vi "Shooter Controller.vi"(8 "error in":errorcluster) -> ()   [LabVIEW 2019]
doc: "This VI executes continuously carrying out the current operation and responding to updates or new operations. It will often contain the timing or control code that is difficult to place directly in TeleOp. This VI generally opens all sensors and motors and isolates the rest of the robot code from knowing how the operations are carried out."
uses:
  <vilib>/Rock Robotics/WPI/Framework/Completion Status.ctl
  Shooter Setpoints.ctl
  Shooter Operations.ctl
  <vilib>/Rock Robotics/WPI/ThirdParty/REV Robotics/SPARK MAX/Typedef/Spark MAX Idle Mode.ctl
  <vilib>/Rock Robotics/WPI/ThirdParty/REV Robotics/SPARK MAX/Typedef/Spark MAX Control Type.ctl
  <vilib>/Rock Robotics/Network Tables/NT Write Boolean.vi
panel:
  in  "Interactive Values":T1
  out "Current\nCmd":string
  in  "Buttons":cluster{"Execute Cmd":bool, "Abort Cmd":bool}
  out "Command Timing":cluster{"Start Time (ms)":u32, "Iterations":i32}
  out "Status":T3
  # "Tip: It may be helpful to observe inputs and sensor values.\nYou may also want to display tuning or debugging controls."
  # "Interactive Command: You may fill in the settings for a command\nand schedule it with the Execute button. You can observe and abort\nany command while fine tuning the code for the controller."
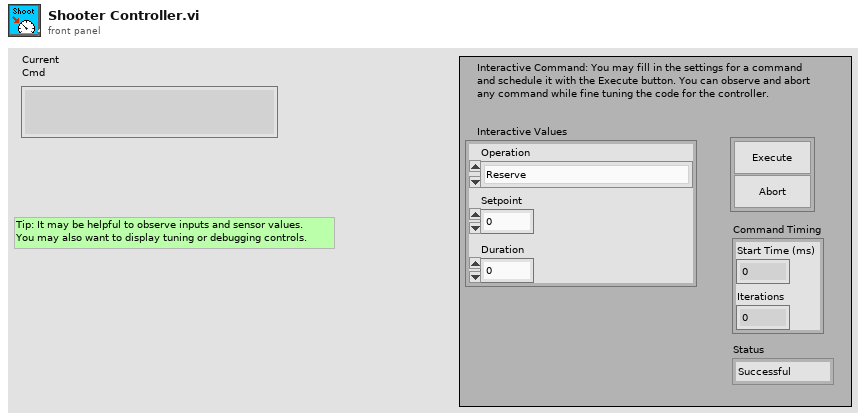
[diagram p1: front panel]
types:
  T1 = typedef "Shooter Setpoints.ctl" = cluster{"Operation":T2, "Setpoint":dbl, "Duration":dbl}
  T2 = typedef "Shooter Operations.ctl" = enum16{"Reserve", "Read Current", "Immediate", "Shoot for Time"}
  T3 = typedef "Completion Status.ctl" = enum16{"Successful", "Aborted", "Incomplete"}
  T4 = typedef "Spark MAX Idle Mode.ctl" = enum16{"Coast", "Brake"}
  T5 = typedef "WPI_MotorControlDeviceRef.ctl" = cluster{"DeviceStatus":errorcluster, "Type":T6, "PWM":cluster{"PWM Channel":T7, "DeadBand":T8}, "CAN":cluster{"Device Number":u8, "SetOutput VI Ref":variant, "GetOutput VI Ref":variant, "Enable VI Ref":variant, "Disable VI Ref":variant, "Data":variant}, "Invert":bool, "DIO PWM":cluster{"PWM \"Enable\" Channel":T7, "DIOChannel":T9, "PWM Rate":dbl}}
  T6 = typedef "WPI_MotorControlType.ctl" = enum16{"PWM", "CAN", "DIO PWM"}
  T7 = typedef "FPGA_DIOPWMChannel.ctl" = enum8{"PWM 0", "PWM 1", "PWM 2", "PWM 3", "PWM 4", "PWM 5", "PWM 6", "PWM 7", "PWM 8", "PWM 9", "PWM MXP 0", "PWM MXP 1", "PWM MXP 2", "PWM MXP 3", "PWM MXP 4", "PWM MXP 5", "PWM MXP 6", "PWM MXP 7", "PWM MXP 8", "PWM MXP 9", "Invalid"}
  T8 = typedef "WPI_PWMDeadband.ctl" = cluster{"Name":string, "maxPositivePwm":i32, "minPositivePwm":i32, "centerPwm":i32, "maxNegativePwm":i32, "minNegativePwm":i32, "angularRange":u16}
  T9 = typedef "FPGA_DIOChannel.ctl" = enum8{"DIO 0", "DIO 1", "DIO 2", "DIO 3", "DIO 4", "DIO 5", "DIO 6", "DIO 7", "DIO 8", "DIO 9", "DIO MXP 0", "DIO MXP 1", "DIO MXP 2", "DIO MXP 3", "DIO MXP 4", "DIO MXP 5", "DIO MXP 6", "DIO MXP 7", "DIO MXP 8", "DIO MXP 9", "DIO MXP 10", "DIO MXP 11", "DIO MXP 12", "DIO MXP 13", "DIO MXP 14", "DIO MXP 15", "SPI Port CS1", "SPI Port CS2", "SPI Port CS3", "SPI Port MISO", "SPI Port MOSI", "Invalid"}
  T10 = typedef "Command Status Info.ctl" = cluster{"Name":string, "Status":T3, "notifier out":T11}
  T11 = typedef "Completion Notifier.ctl" = refnum<notifier>
  T12 = cluster{"Current Command":T1, "Command Timing":cluster{"Start Time (ms)":u32, "Iterations":i32}, "Command Arguments":cluster{"Command Info":T10, "Description":string, "Default Command":T1, "queue out":refnum<queue>, "Subsystem Name":string}}
  T13 = typedef "Spark MAX Control Type.ctl" = enum16{"Percent VBus", "Voltage", "Velocity", "Position", "Smart Motion", "Current", "Smart Velocity"}
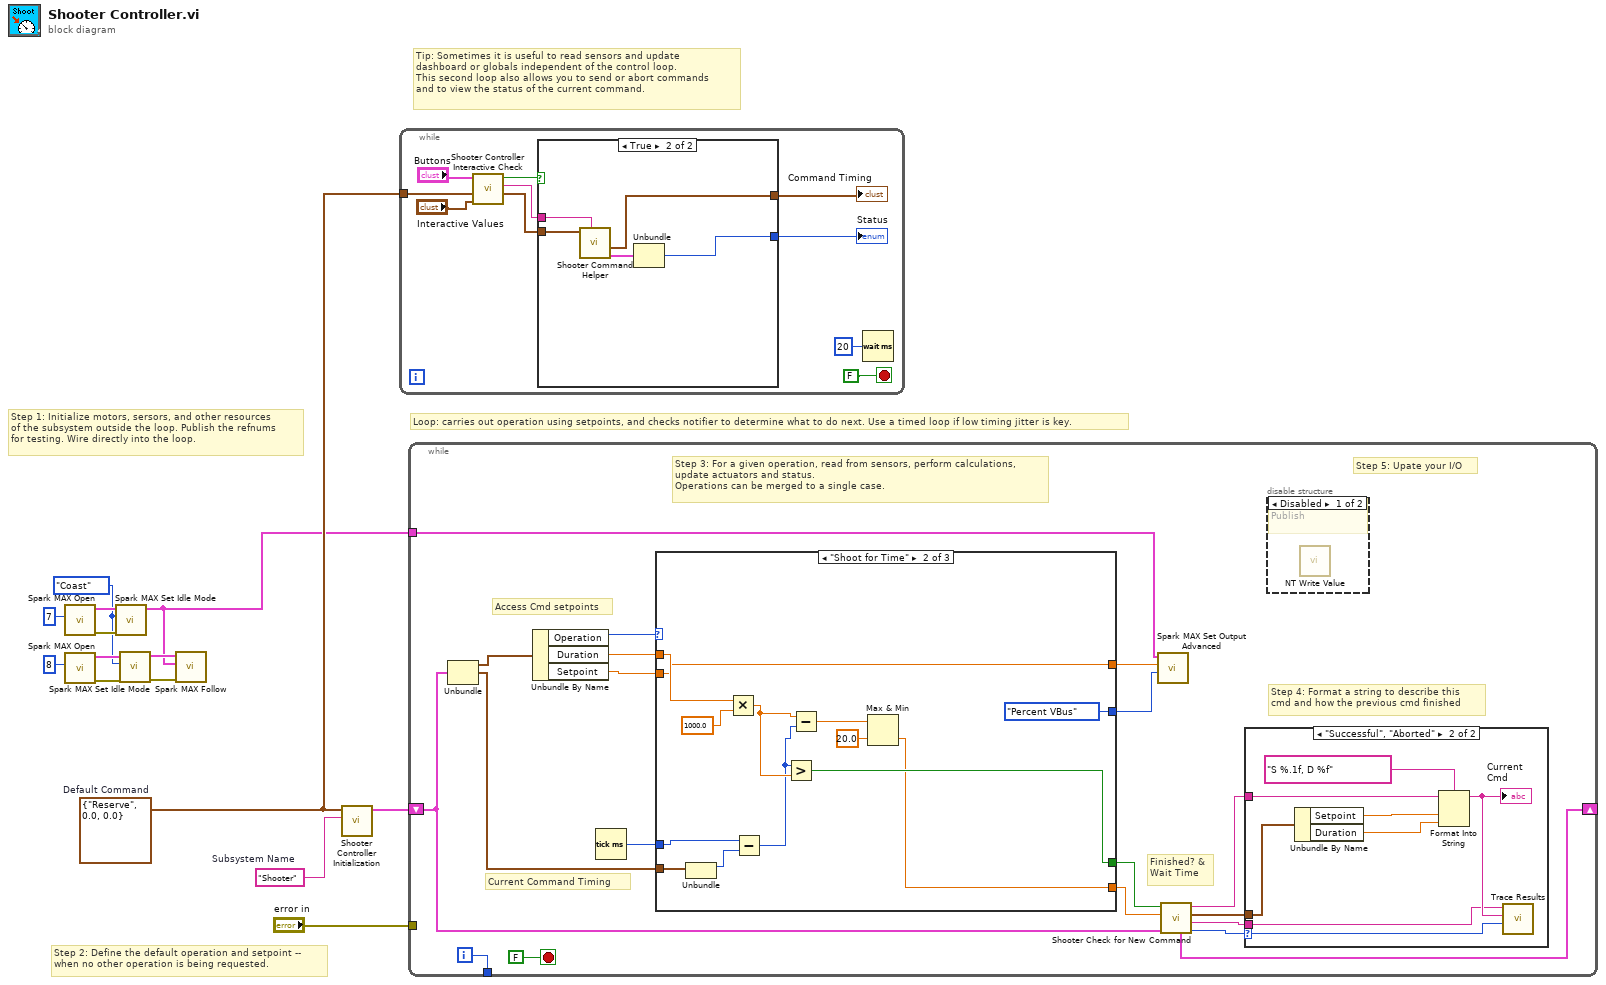
[diagram p0: block diagram]
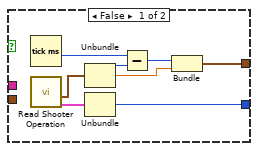
[diagram p2: hidden frame]
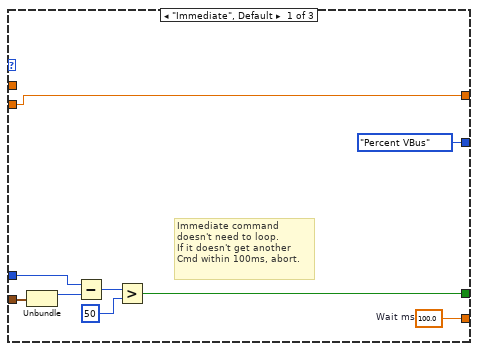
[diagram p5: hidden frame]
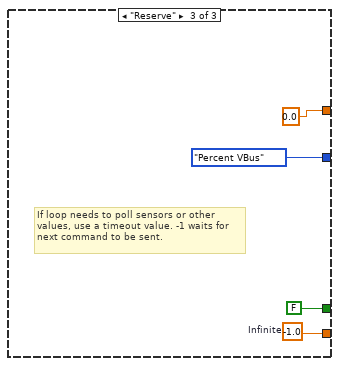
[diagram p6: hidden frame]
diagram:
  w6 = Spark_MAX_Idle_Mode."Coast" ("Idle Mode")
  w11 = T1 {"Operation"=enum."Reserve", "Setpoint"=0.0, "Duration"=0.0}  # Default Command
  w12 = "Shooter"  # Subsystem Name
  # "Tip: Sometimes it is useful to read sensors and update\ndashboard or globals independent of the control loop.\nThis second loop also allows you to send or abort commands\nand to view the status of the current command."
  # "Step 2: Define the default operation and setpoint --\nwhen no other operation is being requested."
  # "Step 1: Initialize motors, sersors, and other resources\nof the subsystem outside the loop. Publish the refnums\nfor testing. Wire directly into the loop."
  # "Loop: carries out operation using setpoints, and checks notifier to determine what to do next. Use a timed loop if low timing jitter is key."
  n1 = call <vilib>:"Spark MAX Open.vi"("Device Number"=u8 7) -> ("error out"=w10:errorcluster, "MotorControlDeviceRef"=w9:T5)  [unwired: 9 in]
  n2 = call <vilib>:"Spark MAX Open.vi"("Device Number"=u8 8) -> ("error out"=w7:errorcluster, "MotorControlDeviceRef"=w8:T5)  [unwired: 9 in]
  n3 = call <vilib>:"Spark MAX Set Idle Mode.vi"("error in (no error)"=w10, "Idle Mode"=w6, "MotorControlDeviceRef in"=w9) -> ("MotorControlDeviceRef out"=w1:T5)  [unwired: 7 in, 1 out]
  n4 = call <vilib>:"Spark MAX Set Idle Mode.vi"("error in (no error)"=w7, "Idle Mode"=w6, "MotorControlDeviceRef in"=w8) -> ("error out"=w3:errorcluster, "MotorControlDeviceRef out"=w2:T5)  [unwired: 7 in]
  n5 = call <vilib>:"Spark MAX Follow.vi"("error in (no error)"=w3, "Master Controller"=w1, "MotorControlDeviceRef"=w2) -> ()  [unwired: 7 in, 2 out]
  n6 = call "Shooter Controller Initialization.vi"("Subsystem Name"=w12, "Default Command"=w11) -> ("Current Command"=w13:T12)  [unwired: 9 in]
  n7 = while {
    tunnel: w11 -> [w21]
    stop <- FALSE stop-if-true
    n8 = call "Shooter Controller Interactive Check.vi"("Interactive Command in"="Interactive Values", "Default Command"=w21, "Buttons"="Buttons") -> ("Interactive Command out"=w18:T1, "Trace String"=w19:string, "Schedule"=w20:bool)  [unwired: 6 in]
    n9 = case shown="True" w20 {
      tunnel: [w32 w37] -> w17
      tunnel: w18 -> [_ w35]
      tunnel: [w28 w33] -> w16
      tunnel: w19 -> [_ w36]
      frame False {
        n10 = Tick Count (ms)() -> (millisecond timer value=w27:u32)
        n11 = call "Read Shooter Operation.vi"() -> ("Command Info"=w25:T10, "SubSystem Data"=w26:T1)  [unwired: 9 in, 1 out]
        n12 = Unbundle(w26) -> ("Operation"=w31:T2, "Setpoint"=w29:dbl)  [unwired: 1 out]
        n13 = Unbundle(w25) -> ("Status"=w32:T3)  [unwired: 2 out]
        n14 = Subtract(x=w27, y=w31) -> (x-y=w30:u32)
        n15 = Bundle(w30, "Setpoint"=w29) -> (w28:cluster{u32, "Setpoint":dbl})  [unwired: 1 in]
      }
      frame True {
        n16 = call "Shooter Command Helper.vi"("Description"=w36, "SubSystem Data"=w35) -> ("Command Info Out"=w34:T10, "Command Timing"=w33:cluster{"Start Time (ms)":u32, "Iterations":i32})  [unwired: 7 in, 1 out]
        n17 = Unbundle(w34) -> ("Status"=w37:T3)  [unwired: 2 out]
      }
    }
    "Status" <- w17
    "Command Timing" <- w16
    n18 = Wait (ms)(milliseconds to wait=u32 20) -> ()  [unwired: 1 out]
  }
  n19 = while {
    shift-right: [w48] -> _
    shift-left: w13 -> [w41]
    tunnel: [w55] -> _
    tunnel: "error in" -> [_]
    tunnel: w1 -> [w40]
    i -> [w55]
    stop <- FALSE stop-if-true
    # "Step 5: Upate your I/O"
    # "Step 4: Format a string to describe this\ncmd and how the previous cmd finished"
    # "Current Command Timing"
    # "Access Cmd setpoints"
    # "Finished? &\nWait Time"
    # "Step 3: For a given operation, read from sensors, perform calculations,\nupdate actuators and status.\nOperations can be merged to a single case."
    n20 = Unbundle(w41) -> ("Current Command"=w54:T1, "Command Timing"=w50:cluster{"Start Time (ms)":u32, "Iterations":i32})  [unwired: 1 out]
    n21 = Unbundle By Name(w54) -> ("Operation"=w53:T2, "Duration"=w52:dbl, "Setpoint"=w49:dbl)
    n22 = Tick Count (ms)() -> (millisecond timer value=w51:u32)
    n23 = case shown="\"Shoot for Time\"" w53 {
      tunnel: [w73 w76 w90] -> w46
      tunnel: [w67 w81 FALSE ("ignore previous (F)")] -> w47
      tunnel: w50 -> [w69 w86 _]
      tunnel: w52 -> [_ w83 _]
      tunnel: w51 -> [w68 w84 _]
      tunnel: w49 -> [w66 w74 _]
      tunnel: [w66 w74 0.0] -> w39
      tunnel: [Spark_MAX_Control_Type."Percent VBus" ("Control Mode") Spark_MAX_Control_Type."Percent VBus" ("Control Mode") Spark_MAX_Control_Type."Percent VBus" ("Control Mode")] -> w38
      frame "Immediate", Default {
        w73 = 100.0  # Wait ms
        # "Immediate command\ndoesn't need to loop.\nIf it doesn't get another\nCmd within 100ms, abort."
        n24 = Unbundle(w69) -> ("Start Time (ms)"=w72:u32)  [unwired: 1 out]
        n25 = Subtract(x=w68, y=w72) -> (x-y=w71:u32)
        n26 = Greater?(x=w71, y=u8 50 ("Left Motor")) -> (0:w67:bool)
      }
      frame "Shoot for Time" {
        n27 = Unbundle(w86) -> ("Start Time (ms)"=w85:u32)  [unwired: 1 out]
        n28 = Multiply(x=w83, y=1000.0) -> (x*y=w80:dbl)
        n29 = Subtract(x=w84, y=w85) -> (x-y=w79:u32)
        n30 = Greater?(x=w79, y=w80) -> (0:w81:bool)
        n31 = Subtract(x=w80, y=w79) -> (x-y=w78:dbl)
        n32 = Max & Min(x=w78, y=20.0) -> (min(x,y)=w76:dbl)  [unwired: 1 out]
      }
      frame "Reserve" {
        w90 = -1.0  # Infinite
        # "If loop needs to poll sensors or other\nvalues, use a timeout value. -1 waits for\nnext command to be sent."
      }
    }
    n33 = call <vilib>:"Spark MAX Set Output Advanced.vi"("Control Mode"=w38, "Setpoint"=w39, "MotorControlDevRef"=w40) -> ()  [unwired: 7 in, 2 out]
    n34 = call "Shooter Check for New Command.vi"("Current Command"=w41, "Wait time (ms)"=w46, "Finished?"=w47) -> ("Completion"=w42:T3, "Subsystem Name"=w43:string, "Current Command"=w44:T1, "Initial Trace String"=w45:string, "NextCommand"=w48:T12)  [unwired: 4 in]
    n35 = case shown="\"Successful\", \"Aborted\"" w42 {
      selector: w42 -> [_ w64]
      tunnel: w45 -> [_ w60]
      tunnel: w44 -> [_ w61]
      tunnel: w43 -> [_ w57]
      frame "Incomplete", Default {
        # "Continuing current command"
      }
      frame "Successful", "Aborted" {
        # "Report and setup for next command"
        n36 = Unbundle By Name(w61) -> ("Setpoint"=w63:dbl, "Duration"=w58:dbl)
        n37 = Format Into String(format string="S %.1f, D %f", initial string=w60, w63, w58) -> (resulting string=w59:string)  [unwired: 1 in, 1 out]
        "Current\nCmd" <- w59
        n38 = call <vilib>:"Trace Results.vi"("Status of previous command"=w64, "Description"=w59, "Subsystem"=w57) -> ()  [unwired: 9 in]
      }
    }
    n39 = disable-structure shown="Disabled" {
      frame Disabled {
        # "Publish"
        n40 = call-poly <vilib>:"NT Write Value.vi"() -> ()  [unwired: 11 in, 1 out]
      }
      frame Enabled {
      }
    }
  }
